vi "BuildClass.vi"(6 "BuildPath":path, 7 "Parent":enum16{"None", "Interface", "Class"}(ring)=enum."Interface", 8 "error in (no error)":errorcluster, 9 "This Application":refnum<vi>, 10 "ParentRef":refnum<vi>, 11 "Interface in":refnum<class "Interface.lvclass">) -> (0 "error out":errorcluster, 3 "Interface out":refnum<class "Interface.lvclass">)   [LabVIEW 2020, in "Mermaid.lvlib" / "Interface.lvclass"]
uses:
  Interface.lvclass
  Interface.lvclass/Interface.ctl
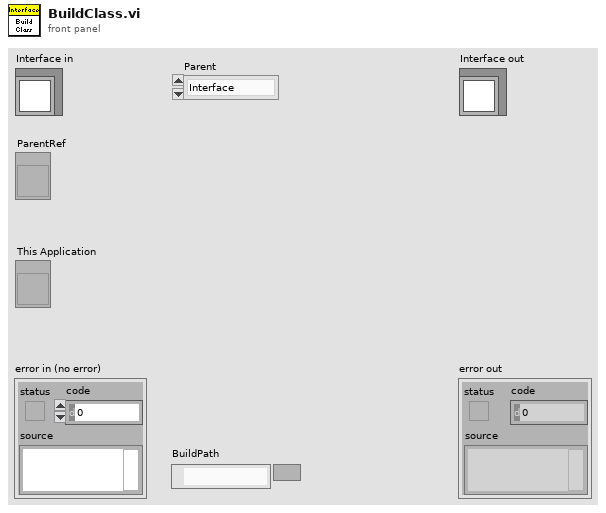
[diagram p1: front panel]
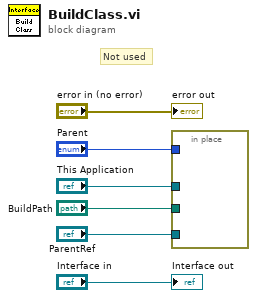
[diagram p0: block diagram]
diagram:
  # "Not used"
  n1 = in-place {
    in-place-border: "ParentRef" -> [_]
    in-place-border: "This Application" -> [_]
    in-place-border: "Parent" -> [_]
    in-place-border: "BuildPath" -> [_]
  }
  "error out" <- "error in (no error)"
  "Interface out" <- "Interface in"
